vi "Dequeue Command.vi"(7 "Wait? (T)":bool=TRUE, 8 "error in (no error)":errorcluster, 11 "TCP Client in":refnum<class "TCP Client.lvclass">) -> (0 "error out":errorcluster, 1 "timed out?":bool, 2 "Command":T1, 3 "TCP Client out":refnum<class "TCP Client.lvclass">)   [LabVIEW 2012, in "Stream-TCP.lvlib" / "TCP Client.lvclass"]
uses:
  TCP Client.lvclass
  Client Command.ctl
  Stream-TCP.lvlib
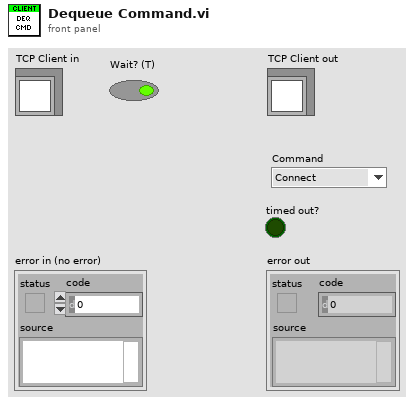
[diagram p1: front panel]
types:
  T1 = typedef "Stream-TCP.lvlib/Client Command.ctl" = enum16{"Connect", "Close", "Shutdown", "Reconnect"}
  T2 = typedef "Stream-TCP.lvlib/Client Command Queue.ctl" = refnum<queue>
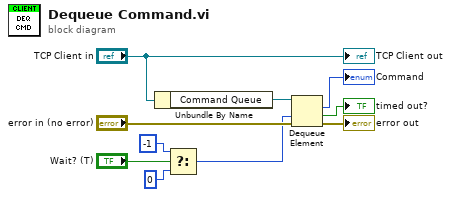
[diagram p0: block diagram]
diagram:
  n1 = Unbundle By Name("TCP Client in") -> ("Command Queue"=w9:T2)
  n2 = Select(t=-1, s="Wait? (T)", f=0) -> (s? t:f=w3:i32)
  n3 = Dequeue Element(queue=w9, timeout in ms (-1)=w3, error in (no error)="error in (no error)") -> (element=→"Command":T1, timed out?=→"timed out?":bool, error out=→"error out":errorcluster)  [unwired: 1 out]
  "TCP Client out" <- "TCP Client in"
